vi "Get Connection Reference (TCP).vi"(8 "error in":errorcluster, 11 "connection info in":T1) -> (0 "error out":errorcluster, 2 "connection ID out":refnum<k5>, 3 "connection info out":T1)   [LabVIEW 2013, in "NI STM.lvlib"]
doc: "Returns the TCP/IP connection reference."
uses:
  NI STM.lvlib
  TCP Connection Info.ctl
  SubVIs/MetaDataElement.ctl
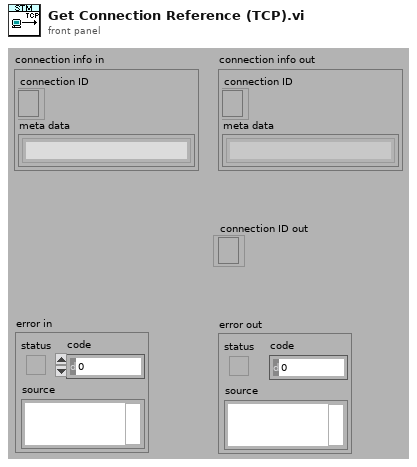
[diagram p1: front panel]
types:
  T1 = typedef "NI STM.lvlib/TCP Connection Info.ctl" = cluster{"connection ID":refnum<k5>, "meta data":T2[]}
  T2 = typedef "NI STM.lvlib/MetaDataElement.ctl" = string
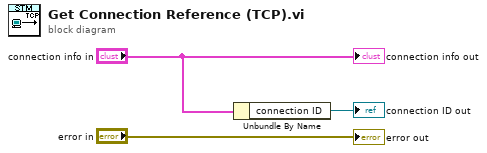
[diagram p0: block diagram]
diagram:
  n1 = Unbundle By Name("connection info in") -> ("connection ID"=→"connection ID out":refnum<k5>)
  "connection info out" <- "connection info in"
  "error out" <- "error in"
